vi "Read Serialized.vi"(8 "error in (no error)":errorcluster, 11 "FM Sweep in":refnum<class "FM Sweep.lvclass">) -> (0 "error out":errorcluster, 2 "Serialized":T1, 3 "FM Sweep out":refnum<class "FM Sweep.lvclass">)   [LabVIEW 2020, in "FM Sweep.lvclass"]
uses:
  FM Sweep.lvclass
  Serialized.ctl
  FM Sweep.lvclass/FM Sweep.ctl
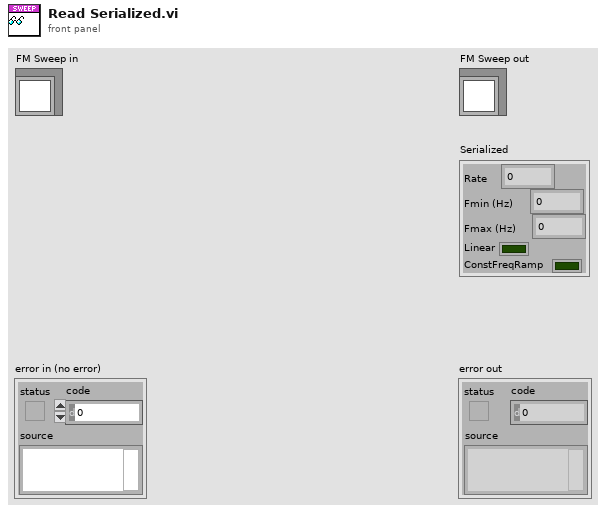
[diagram p1: front panel]
types:
  T1 = typedef "FM Sweep.lvclass/Serialized.ctl" = cluster{"Rate":dbl, "Fmin (Hz)":dbl, "Fmax (Hz)":dbl, "Linear":bool, "ConstFreqRamp":bool}
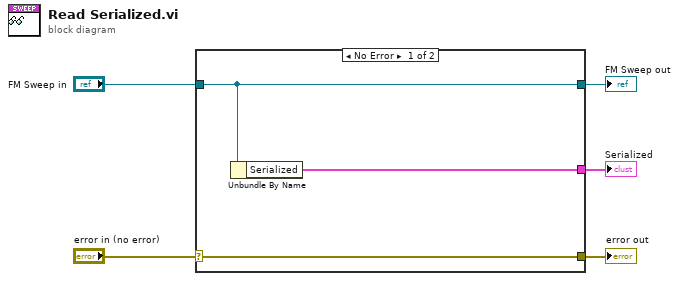
[diagram p0: block diagram]
diagram:
  n1 = case shown="No Error" "error in (no error)" {
    selector: "error in (no error)" -> [w8 w9]
    tunnel: [w8 w9] -> w4
    tunnel: [w7 w10] -> w2
    tunnel: "FM Sweep in" -> [w7 w10]
    tunnel: [w6 _] -> w1
    frame No Error {
      n2 = Unbundle By Name(w7) -> ("Serialized"=w6:T1)
    }
    frame Error {
    }
  }
  "error out" <- w4
  "FM Sweep out" <- w2
  "Serialized" <- w1
